vi "Calculate Projection Matrix.vi"(10 "Camera":T1, 11 "Screen Dimensions":T2) -> (3 "Projection Matrix":sgl[][](array[numeric]))   [LabVIEW 2020, in "3D.lvlib"]
uses:
  3D.lvlib
  Raster/Screen Dimensions.ctl
  Camera.ctl
  Raster/Raster.lvlib
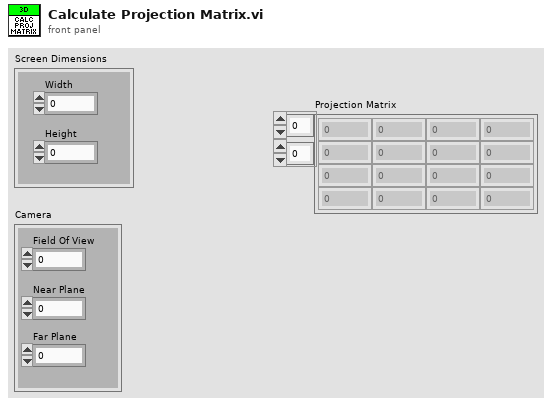
[diagram p1: front panel]
types:
  T1 = typedef "3D.lvlib/Camera.ctl" = cluster{"Field Of View":sgl, "Near Plane":sgl, "Far Plane":sgl}
  T2 = typedef "Raster.lvlib/Screen Dimensions.ctl" = cluster{"Width":u32, "Height":u32}
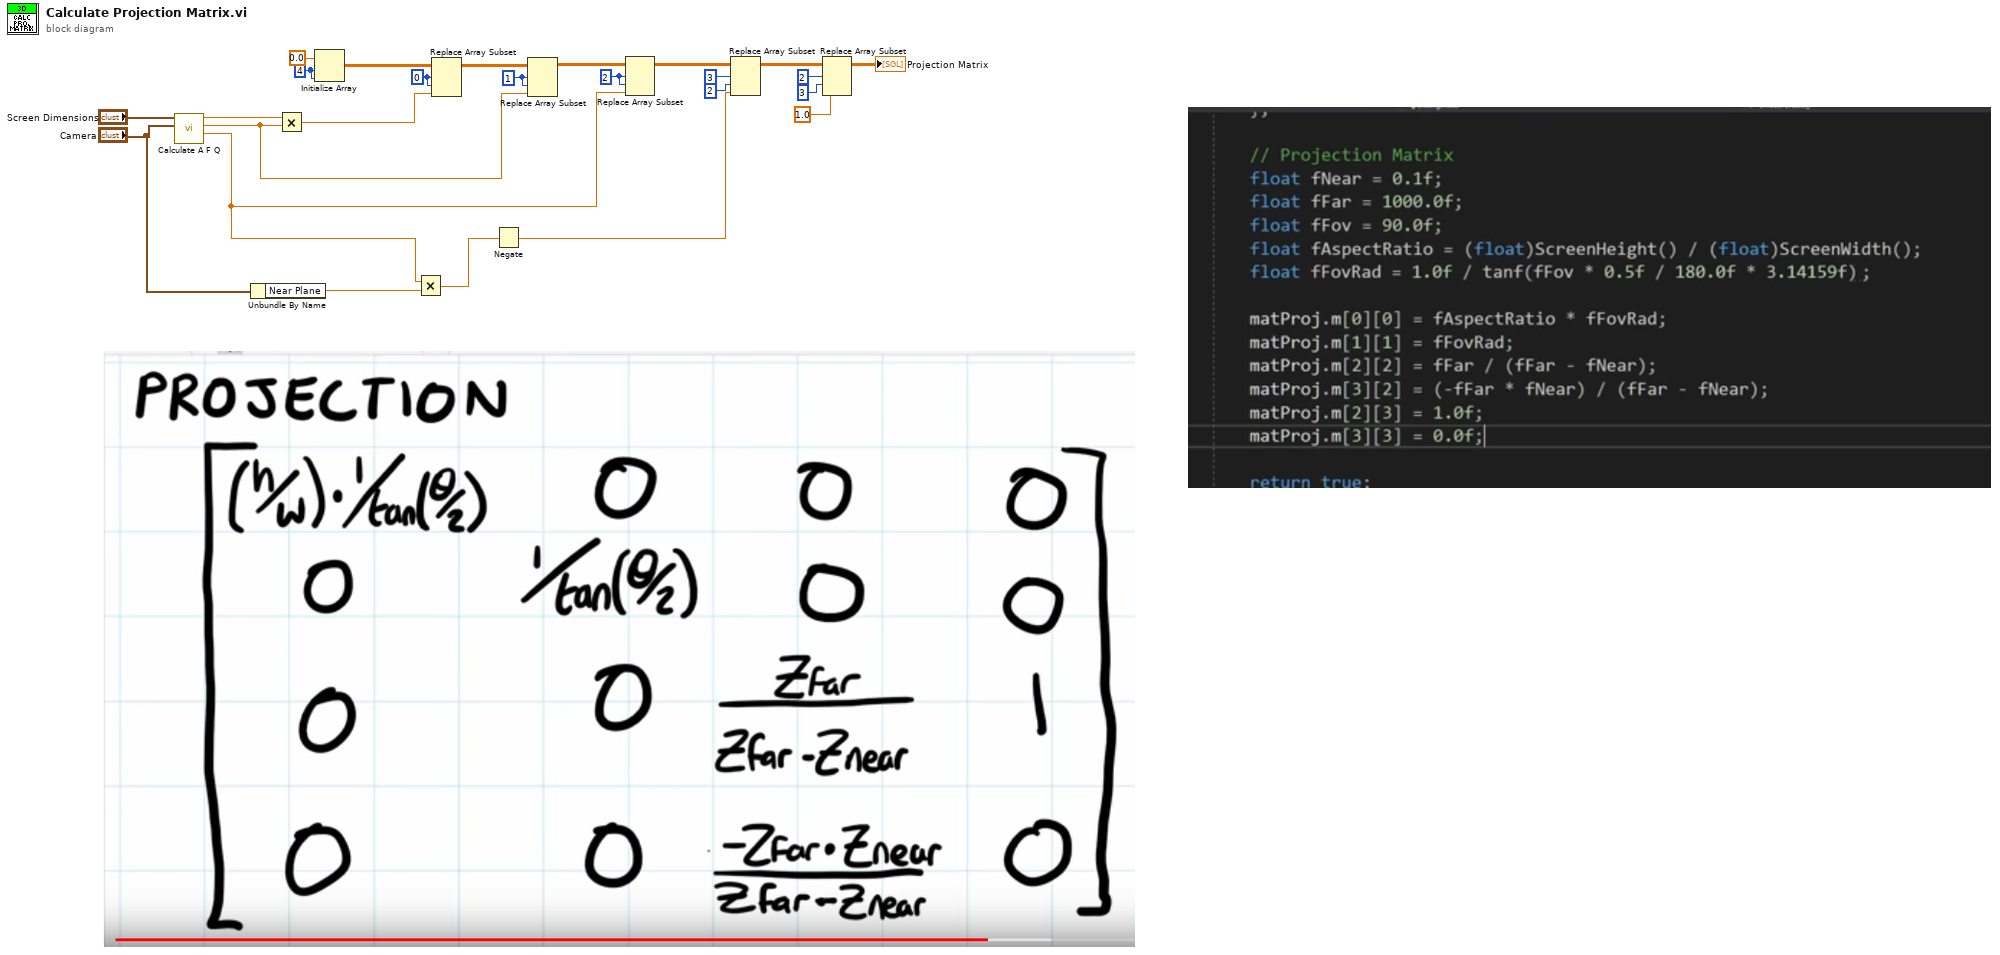
[diagram p0: block diagram]
diagram:
  w19 = 2 ("index (row)")
  w20 = 1 ("index (row)")
  w22 = 0 ("index (row)")
  w24 = 4 ("dimension size")
  n1 = call "Calculate A F Q.vi"("Camera"="Camera", "Screen Dimensions"="Screen Dimensions") -> ("q"=w2:sgl, "f"=w7:sgl, "Aspect Ratio"=w9:sgl)  [unwired: 7 in]
  n2 = Unbundle By Name("Camera") -> ("Near Plane"=w3:sgl)
  n3 = Multiply(x=w9, y=w7) -> (x*y=w8:sgl)
  n4 = Initialize Array(sgl 0.0 ("element"), w24, w24) -> (w23:sgl[][])
  n5 = Multiply(x=w2, y=w3) -> (x*y=w1:sgl)
  n6 = Replace Array Subset(array=w23, new element=w8, index (row)=w22, index (col)=w22) -> (w21:sgl[][])
  n7 = Negate(x=w1) -> (-x=w6:sgl)
  n8 = Replace Array Subset(array=w21, new element=w7, index (row)=w20, index (col)=w20) -> (w18:sgl[][])
  n9 = Replace Array Subset(array=w18, new element=w2, index (row)=w19, index (col)=w19) -> (w16:sgl[][])
  n10 = Replace Array Subset(array=w16, new element=w6, index (row)=3, index (col)=2 ("index (row)")) -> (w12:sgl[][])
  n11 = Replace Array Subset(array=w12, new element=sgl 1.0 ("new element/subarray"), index (row)=2, index (col)=3 ("index (row)")) -> (→"Projection Matrix":sgl[][])
